vi "Get Max Cell Capacity.vi"(11 "error in (no error)":errorcluster) -> (4 "Max Capacity[]":i32[](array[numeric]), 15 "error out":errorcluster)   [LabVIEW 2014, in "Dragon Tamers.lvlib"]
uses:
  Dragon Tamers.lvlib
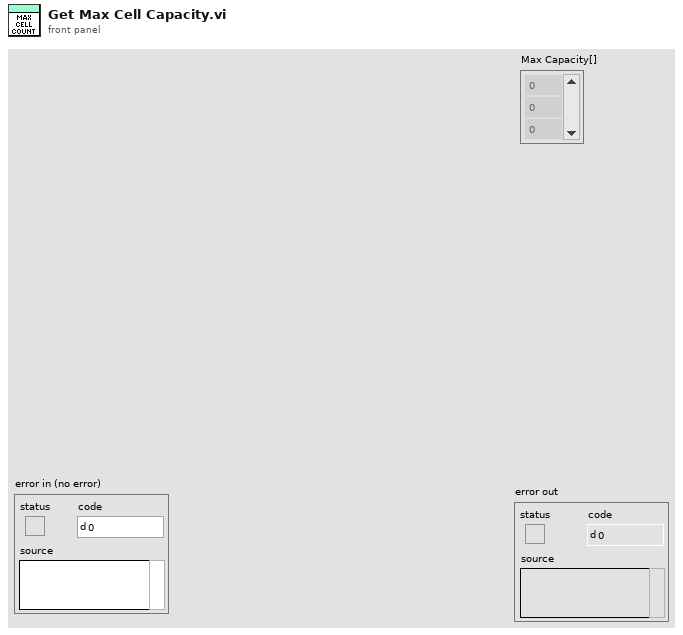
[diagram p1: front panel]
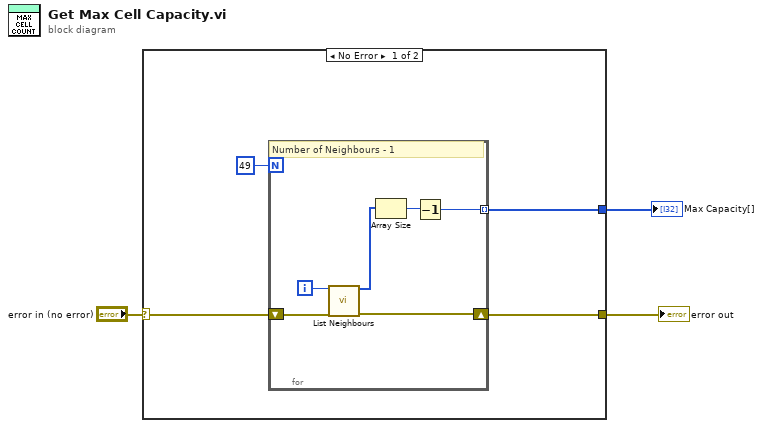
[diagram p0: block diagram]
diagram:
  n1 = case shown="No Error" "error in (no error)" {
    selector: "error in (no error)" -> [w7 w14]
    tunnel: [w5 w14] -> w2
    tunnel: [w4 _] -> w1
    frame No Error {
      n2 = for {
        N: 49 -> [_]
        tunnel: [w9] -> w4 mode=indexing
        shift-right: [w8] -> w5
        shift-left: w7 -> [w13]
        i -> [w12]
        # "Number of Neighbours - 1"
        n3 = call "List Neighbours.vi"("Cell Index"=w12, "error in (no error)"=w13) -> ("Neighbours"=w11:i32[], "error out"=w8:errorcluster)  [unwired: 11 in, 1 out]
        n4 = Array Size(array=w11) -> (size(s)=w10:i32)
        n5 = Decrement(x=w10) -> (x-1=w9:i32)
      }
    }
    frame Error {
    }
  }
  "error out" <- w2
  "Max Capacity[]" <- w1
